vi "Run In Test.vi"(8 "error in (no error)":errorcluster, 10 "Model in":refnum<class "Model.lvclass">, 11 "Test Actuator State in":refnum<class "Test Actuator State.lvclass">) -> (0 "error out":errorcluster, 2 "Model out":refnum<class "Model.lvclass">, 3 "Test Actuator State out":refnum<class "Test Actuator State.lvclass">)   [LabVIEW 2016, in "Test Actuator State.lvclass"]
uses:
  Test Actuator State.lvclass
  Model/Model/Model.lvclass
  Typedefs/TestStatus.ctl
  Model/Model/Model.lvclass/Model.ctl
  Typedefs/FAMT Typedefs.lvlib
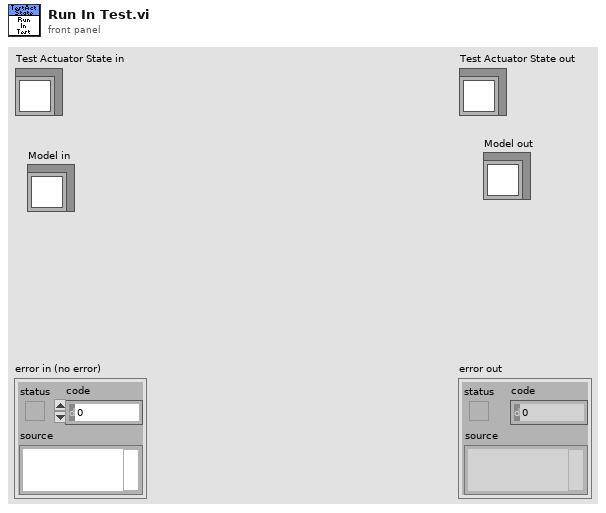
[diagram p1: front panel]
types:
  T1 = typedef "FAMT Typedefs.lvlib/TestStatus.ctl" = enum16{"Not Run", "Running", "Passed", "Failed"}
  T2 = typedef "FAMT Typedefs.lvlib/AllTestStatus.ctl" = cluster{"Differential Pressure Release Valve Test":T1, "Force Accuracy Test":T1, "Full Force Test":T1, "Operational Force Test":T1, "Sentran Accuracy Test":T1, "Slewing Test":T1, "Tracking Test":T1, "Zero Force Test":T1, "Run In Test":T1}
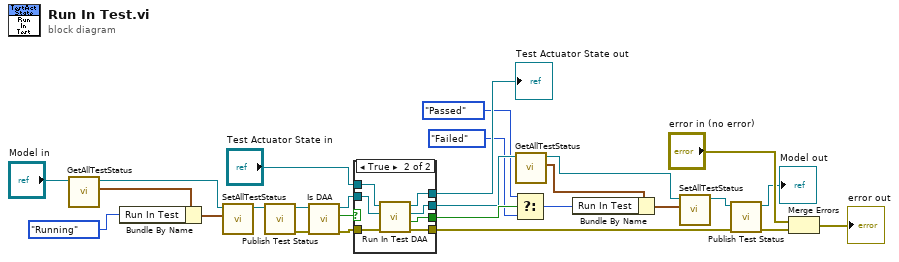
[diagram p0: block diagram]
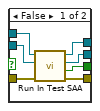
[diagram p2: hidden frame]
diagram:
  n1 = call "GetAllTestStatus.vi"("Model in"="Model in") -> ("AllTestStatus"=w18:T2, "Model out"=w11:refnum<class "Model.lvclass">)  [unwired: 9 in]
  n2 = Bundle By Name(cluster=w18, "Run In Test"=TestStatus."Running" ("Full Force Test")) -> (w17:T2)
  n3 = call "SetAllTestStatus.vi"("AllTestStatus"=w17, "Model in"=w11) -> ("Model out"=w10:refnum<class "Model.lvclass">)  [unwired: 9 in]
  n4 = call "Publish Test Status.vi"("Model in"=w10) -> ("error out"=w8:errorcluster, "Model out"=w9:refnum<class "Model.lvclass">)  [unwired: 9 in]
  n5 = call "Is DAA.vi"("error in (no error)"=w8, "Model in"=w9) -> ("error out"=w21:errorcluster, "IsDAA"=w25:bool, "Model out"=w24:refnum<class "Model.lvclass">)  [unwired: 7 in]
  n6 = case shown="True" w25 {
    tunnel: w24 -> [w32 w41]
    tunnel: "Test Actuator State in" -> [w34 w40]
    tunnel: [w33 w39] -> w22
    tunnel: [w31 w38] -> w12
    tunnel: w21 -> [w30 w37]
    tunnel: [w29 w36] -> w6
    tunnel: [w28 w35] -> w20
    frame False {
      n7 = call "Run In Test SAA.vi"("error in (no error)"=w30, "Model in"=w32, "Test Actuator State in"=w34) -> ("error out"=w29:errorcluster, "Pass"=w28:bool, "Model out"=w31:refnum<class "Model.lvclass">, "Test Actuator State out"=w33:refnum<class "Test Actuator State.lvclass">)  [unwired: 5 in]
    }
    frame True {
      n8 = call "Run In Test DAA.vi"("error in (no error)"=w37, "Model in"=w41, "Test Actuator State in"=w40) -> ("error out"=w36:errorcluster, "Pass"=w35:bool, "Model out"=w38:refnum<class "Model.lvclass">, "Test Actuator State out"=w39:refnum<class "Test Actuator State.lvclass">)  [unwired: 5 in]
    }
  }
  "Test Actuator State out" <- w22
  n9 = Select(t=TestStatus."Passed" ("Full Force Test"), s=w20, f=TestStatus."Failed" ("Full Force Test")) -> (s? t:f=w5:T1)
  n10 = call "GetAllTestStatus.vi"("Model in"=w12) -> ("AllTestStatus"=w15:T2, "Model out"=w13:refnum<class "Model.lvclass">)  [unwired: 9 in]
  n11 = Bundle By Name(cluster=w15, "Run In Test"=w5) -> (w14:T2)
  n12 = call "SetAllTestStatus.vi"("AllTestStatus"=w14, "Model in"=w13) -> ("Model out"=w7:refnum<class "Model.lvclass">)  [unwired: 9 in]
  n13 = call "Publish Test Status.vi"("error in (no error)"=w6, "Model in"=w7) -> ("error out"=w2:errorcluster, "Model out"=→"Model out":refnum<class "Model.lvclass">)  [unwired: 8 in]
  n14 = Merge Errors("error in (no error)", w2) -> (→"error out":errorcluster)
